vi "Open_Instr.vi"(8 "error in (no error)":errorcluster caption="entrée d'erreur (pas d'erreur)", 11 "Class Multimeter (Default) en entrée":refnum<class "Class Instrument Patterm_Matching.lvclass">) -> (0 "error out":errorcluster caption="sortie d'erreur", 3 "Class Multimeter (Default) en sortie":refnum<class "Class Instrument Patterm_Matching.lvclass">)   [LabVIEW 2020, in "Library Instrument & Equipement.lvlib" / "Library Instruments.lvlib" / "Class Instrument Patterm_Matching.lvclass"]
doc: "Opens and acquires an instrument"
uses:
  Class Instrument Patterm_Matching.lvclass
  Class Instrument Patterm_Matching.lvclass/Class Instrument Patterm_Matching.ctl
  Instrument (Default)/Class Instrument (Default).lvclass
  Camera/Class Camera Pattern Matching (Default)/Class Pattern Matching (Default).lvclass
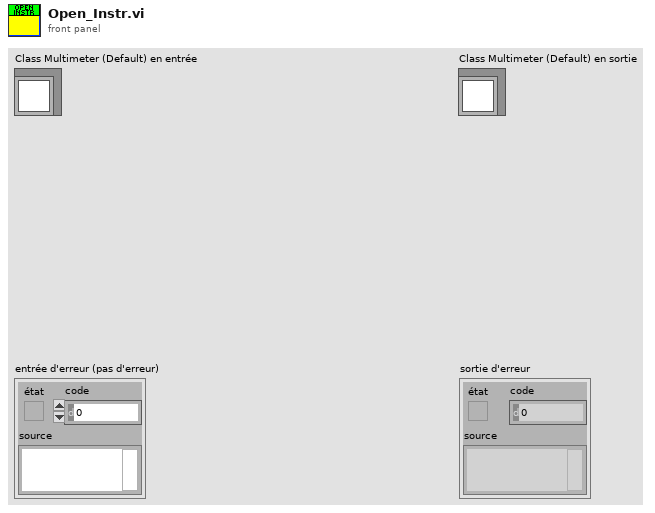
[diagram p1: front panel]
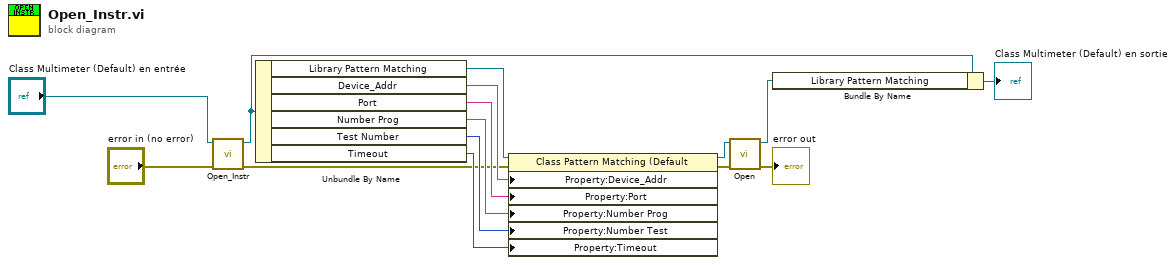
[diagram p0: block diagram]
diagram:
  n1 = call-parent "Open_Instr.vi"("error in (no error)"="error in (no error)", "Class Multimeter (Default) en entrée"="Class Multimeter (Default) en entrée") -> ("error out"=w7:errorcluster, "Class Multimeter (Default) en sortie"=w3:refnum<class "Class Instrument Patterm_Matching.lvclass">)  [unwired: 8 in]
  n2 = Unbundle By Name(w3) -> ("Library Pattern Matching"=w13:refnum<class "Class Pattern Matching (Default).lvclass">, "Device_Addr"=w8:string, "Port"=w9:string, "Number Prog"=w10:string, "Test Number"=w11:u16, "Timeout"=w12:u16)
  n3 = property class="Class Pattern Matching (Default"(reference=w13, error in=w7, "Property:Device_Addr"=w8, "Property:Port"=w9, "Property:Number Prog"=w10, "Property:Number Test"=w11, "Property:Timeout"=w12) -> (reference out=w4:refnum<class "Class Pattern Matching (Default).lvclass">, error out=w5:errorcluster)
  n4 = call-dynamic "Open.vi"("error in (no error)"=w5, "Class Camera IV3-500CA (Default) en entrée"=w4) -> ("error out"=→"error out":errorcluster, "Class Camera IV3-500CA (Default) en Sortie"=w2:refnum<class "Class Pattern Matching (Default).lvclass">)  [unwired: 8 in]
  n5 = Bundle By Name(cluster=w3, "Library Pattern Matching"=w2) -> (→"Class Multimeter (Default) en sortie":refnum<class "Class Instrument Patterm_Matching.lvclass">)
